vi "test.flatten.ClusterCfgTable.vi"() -> ()   [LabVIEW 2017]
uses:
  Configuration/ClusterCfgTable/ClusterCfgTable.lvlib
panel:
  out "error out 2":errorcluster
  out "data 2":T1={"Direction"=enum."Input - 输入", "Group"=1234.0, "Name"=0.245, "PhyChannelCfg"={"Direction"=enum."Input - 输入", "Group"=0.0, "Name"="", "ID"="", "DataType"=enum."1 ___ BOOLEAN", "Protocol"="asdgf", "Description"=""}, "ID"="", "DataType"=enum."0 ___ 没有使用通道", "Protocol"="", "Description"=""}
  out "error out":errorcluster
  in  "PhyChannelCfg":T2={"Direction"=enum."Input - 输入", "Group"=1234.0, "Name"=0.245, "PhyChannelCfg"={"Direction"=enum."Input - 输入", "Group"="1", "Name"="b", "ID"="c", "DataType"=enum."1 ___ BOOLEAN", "Protocol"="asdgf", "Description"="d"}, "ID"="e", "DataType"=enum."0 ___ 没有使用通道", "Protocol"="s", "Description"="s"}
  out "data":T2={"Direction"=enum."Input - 输入", "Group"=1234.0, "Name"=0.245, "PhyChannelCfg"={"Direction"=enum."Input - 输入", "Group"="", "Name"="", "ID"="", "DataType"=enum."1 ___ BOOLEAN", "Protocol"="asdgf", "Description"=""}, "ID"="", "DataType"=enum."0 ___ 没有使用通道", "Protocol"="", "Description"=""}
  out "ConfigStrings":string[](array[string])=["Input - 输入", "1234", "0.245", "Input - 输入", "", "", "", "1 ___ BOOLEAN", "asdgf", "", "", "0 ___ 没有使用通道", "", ""]
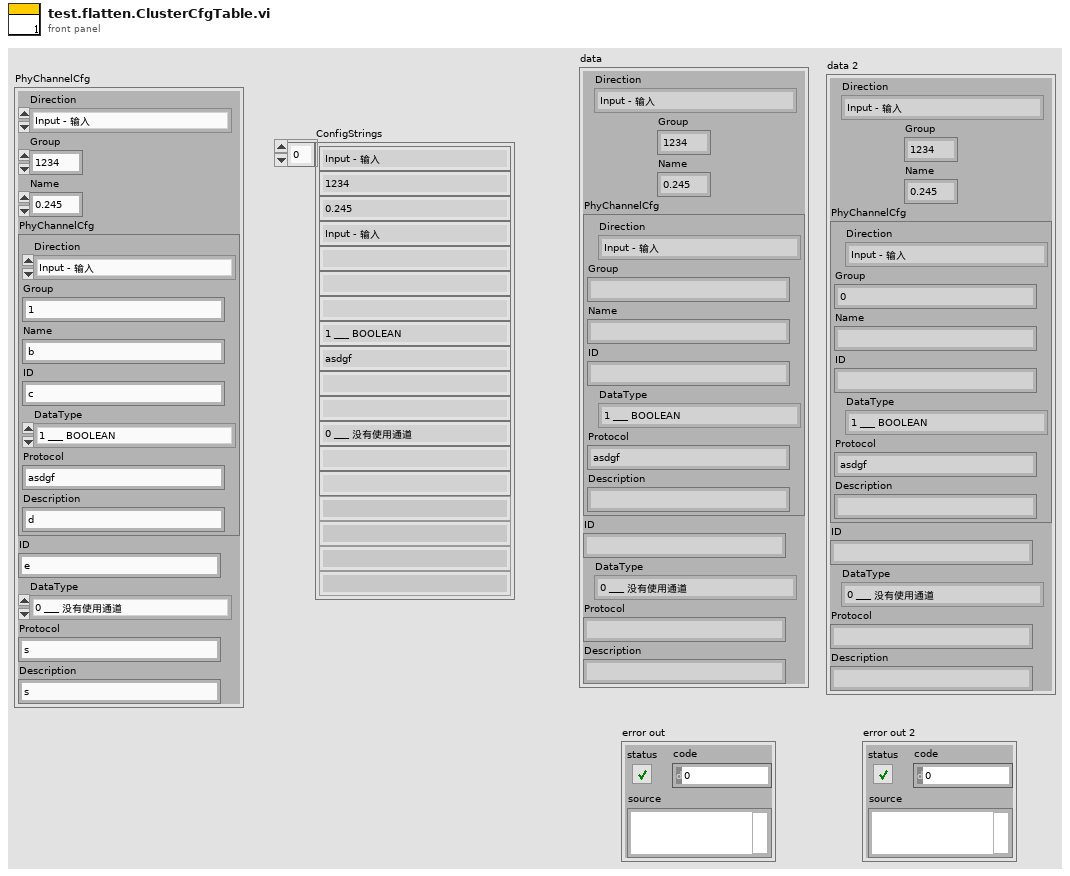
[diagram p1: front panel]
types:
  T1 = cluster{"Direction":enum16{"Input - 输入", "Output - 输出", "Record - 记录"}, "Group":dbl, "Name":dbl, "PhyChannelCfg":cluster{"Direction":enum16{"Input - 输入", "Output - 输出", "Record - 记录"}, "Group":dbl, "Name":string, "ID":string, "DataType":enum16{"0 ___ 没有使用通道", "1 ___ BOOLEAN", "2 ___ U16", "3 ___ DBL"}, "Protocol":string, "Description":string}, "ID":string, "DataType":enum16{"0 ___ 没有使用通道", "1 ___ BOOLEAN", "2 ___ U16", "3 ___ DBL"}, "Protocol":string, "Description":string}
  T2 = cluster{"Direction":enum16{"Input - 输入", "Output - 输出", "Record - 记录"}, "Group":dbl, "Name":dbl, "PhyChannelCfg":cluster{"Direction":enum16{"Input - 输入", "Output - 输出", "Record - 记录"}, "Group":string, "Name":string, "ID":string, "DataType":enum16{"0 ___ 没有使用通道", "1 ___ BOOLEAN", "2 ___ U16", "3 ___ DBL"}, "Protocol":string, "Description":string}, "ID":string, "DataType":enum16{"0 ___ 没有使用通道", "1 ___ BOOLEAN", "2 ___ U16", "3 ___ DBL"}, "Protocol":string, "Description":string}
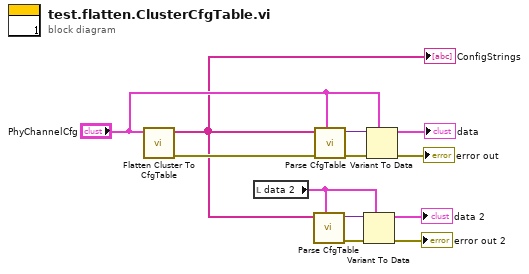
[diagram p0: block diagram]
diagram:
  n1 = call "Flatten Cluster To CfgTable.vi"("Cluster Configuration Typedef"="PhyChannelCfg") -> ("error out"=w8:errorcluster, "CfgTable Row"=w4:string[])  [unwired: 9 in]
  "ConfigStrings" <- w4
  n2 = local read "data 2"() -> (w3:T1)
  n3 = call "Parse CfgTable.vi"("Cluster Configuration Typedef"=w3, "CfgTable Row"=w4) -> ("error out"=w6:errorcluster, "Cluster Configuration Out"=w5:variant)  [unwired: 7 in, 1 out]
  n4 = call "Parse CfgTable.vi"("Cluster Configuration Typedef"="PhyChannelCfg", "error in (no error)"=w8, "CfgTable Row"=w4) -> ("error out"=w11:errorcluster, "Cluster Configuration Out"=w12:variant)  [unwired: 6 in, 1 out]
  n5 = Variant To Data(error in=w6, type=w3, Variant=w5) -> (data=→"data 2":T1, error out=→"error out 2":errorcluster)
  n6 = Variant To Data(error in=w11, type="PhyChannelCfg", Variant=w12) -> (data=→"data":T2, error out=→"error out":errorcluster)
